vi "State_Inc_Button_Hold.vi"(10 "Numeric in":i32, 11 "Floor_Pickup":bool) -> (3 "t":i32)   [LabVIEW 2014]
panel:
  # "Press and hold state\n- This will allow the system to run through its states while a button is pushed\n- Resets states when button is released"
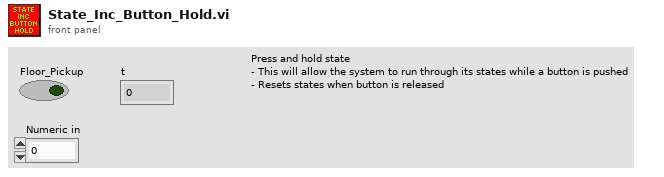
[diagram p1: front panel]
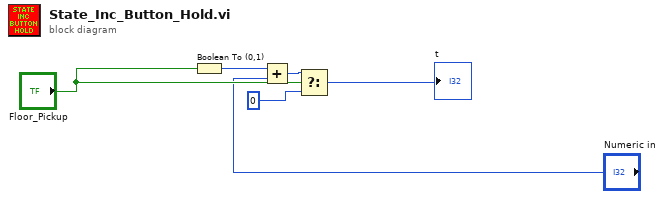
[diagram p0: block diagram]
diagram:
  n1 = Boolean To (0,1)(Boolean="Floor_Pickup") -> (0, 1=w6:i16)
  n2 = Add(x=w6, y="Numeric in") -> (x+y=w1:i32)
  n3 = Select(t=w1, s="Floor_Pickup", f=0 ("t")) -> (s? t:f=→"t":i32)
